vi "ADO Command Set String Parameter Value.vi"(8 "error in (no error)":errorcluster, 9 "String":string, 10 "Index":i32, 11 "ADODB.Parameters":refnum<k7>) -> (0 "error out":errorcluster, 3 "ADODB.Parameters":refnum<k7>)   [LabVIEW 2013]
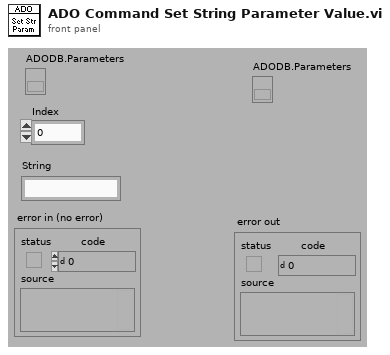
[diagram p1: front panel]
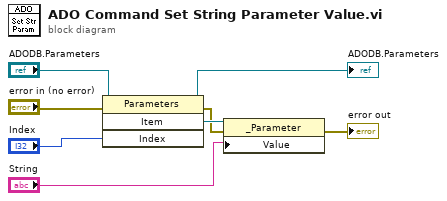
[diagram p0: block diagram]
diagram:
  n1 = invoke class="Parameters" method="Item"(reference="ADODB.Parameters", error in="error in (no error)", "Index"="Index") -> (reference out=→"ADODB.Parameters":refnum<k7>, error out=w7:errorcluster, "Item"=w8:refnum<k7>)  [unwired: 1 in, 1 out]
  n2 = property class="_Parameter"(reference=w8, error in=w7, "Value"="String") -> (error out=→"error out":errorcluster)  [unwired: 1 out]
